vi "Update Chnl Settings.vi"(8 "error in (no error)":errorcluster, 11 "BME_DG_G02 in":refnum<class "BME_DG_G02.lvclass">) -> (0 "error out":errorcluster, 3 "BME_DG_G02 out":refnum<class "BME_DG_G02.lvclass">)   [LabVIEW 2009]
uses:
  BME_DG_G02.lvclass
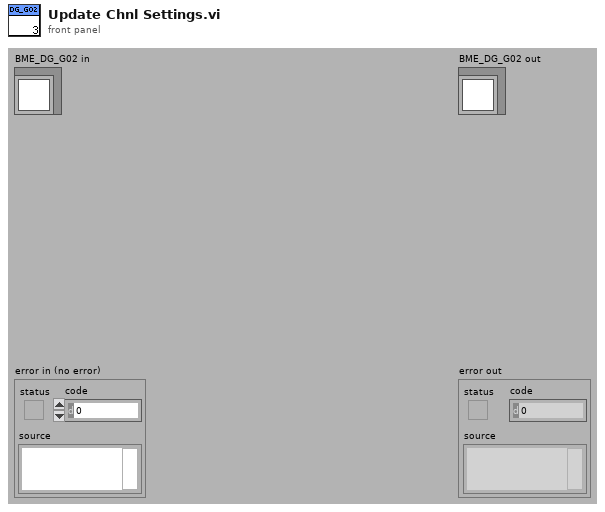
[diagram p1: front panel]
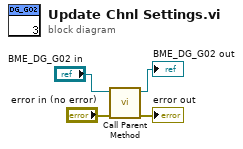
[diagram p0: block diagram]
diagram:
  n1 = call-parent "Call Parent Method"("error in (no error)"="error in (no error)", "BME_DG_Base in"="BME_DG_G02 in") -> ("error out"=→"error out":errorcluster, "BME_DG_Base out"=→"BME_DG_G02 out":refnum<class "BME_DG_G02.lvclass">)  [unwired: 8 in]
